vi "Max Bin transfer (single queue).vi"(11 "Enum":enum16{"1", "2", "3", "4"}(ring)) -> (1 "Next state":enum16{"1", "2", "3", "4"}(ring), 3 "END?":bool)   [LabVIEW 2014]
uses:
  <vilib>/rvi/Emulation/niFpgaEmulationIsFPGAContextNoSignature.vi
  <vilib>/rvi/DataTransferAndStorage/Container/Common/niFpgaContainerGetUniqueNameForEmu.vi
  <vilib>/rvi/Memory/Memory_Emulation/niFpgaMemoryEmulationCacheClearOnFirstRun.vi
  <vilib>/rvi/Memory/Memory_Emulation/nirvimemoryEmulationManagerCache_MakeExclusive.vi
  <vilib>/rvi/Memory/Memory_Emulation/niFpgaMemoryEmulationValidateCache.vi
  <vilib>/rvi/Memory/Memory_Emulation/nirvimemoryEmulationManagerCache_InsertValue.vi
  <vilib>/Utility/error.llb/Clear Errors.vi
  <vilib>/rvi/Memory/Memory_Emulation/nirvimemoryEmulationManagerCache_ReleaseExclusive.vi
  <vilib>/rvi/Memory/Memory_Emulation/nirvimemoryEmulationManagerCache_GetValue.vi
  <vilib>/rvi/Memory/Memory_Emulation/nirvimemoryEmulationManagerCache_SetValue.vi
  <vilib>/rvi/Emulation/niFpgaProcessEmulError.vi
  <vilib>/rvi/Emulation/niFpgaSctlEmulationGetInTimedLoop.vi
  <vilib>/rvi/interface/RandomDataEmulation/niFpgaRandomDataHandleErrors.vi
  <vilib>/rvi/DataTransferAndStorage/Container/XNode/niFpgaContainer.xnode
  <vilib>/rvi/DataTransferAndStorage/Register/Emulation/niFpgaRegisterEmulation.vi
  <vilib>/rvi/interface/RandomDataEmulation/nirviRandomDataFpgaReadWriteTemplate.vi
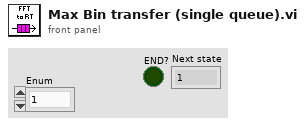
[diagram p1: front panel]
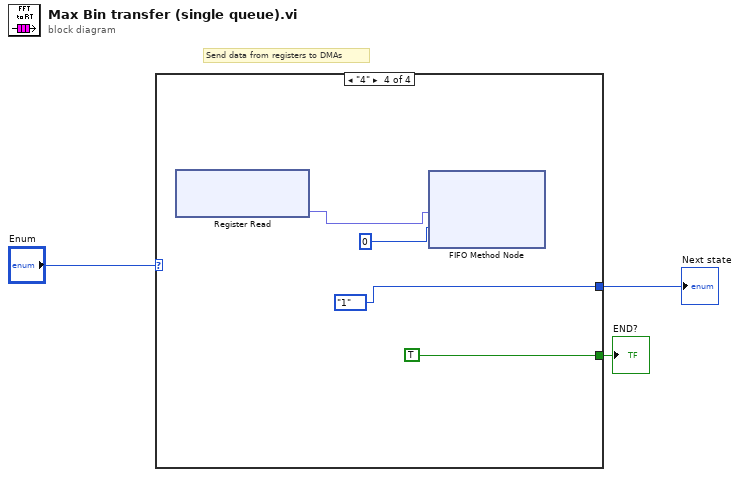
[diagram p0: block diagram]
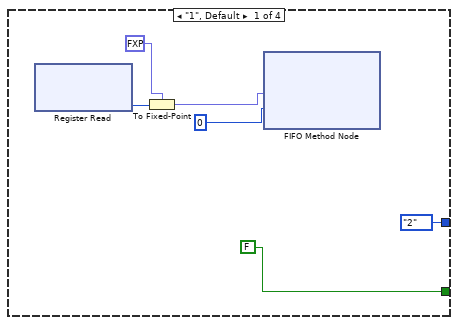
[diagram p2: hidden frame]
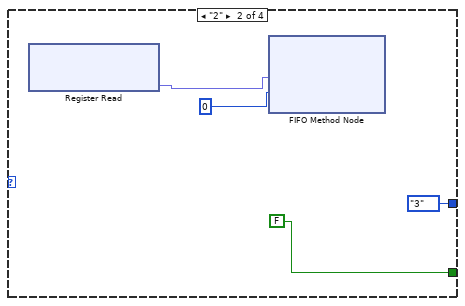
[diagram p3: hidden frame]
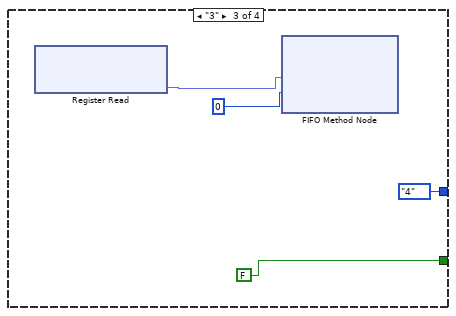
[diagram p4: hidden frame]
diagram:
  # "Send data from registers to DMAs"
  n1 = case shown="\"4\"" "Enum" {
    tunnel: [FALSE ("Timed Out?") FALSE ("Timed Out?") FALSE ("Timed Out?") TRUE ("Timed Out?")] -> w2
    tunnel: [enum16{"1", "2", "3", "4"}."2" ("Enum") enum16{"1", "2", "3", "4"}."3" ("Enum") enum16{"1", "2", "3", "4"}."4" ("Enum") enum16{"1", "2", "3", "4"}."1" ("Enum")] -> w1
    frame "1", Default {
      n2 = xnode ("Register Read")() -> ("Data"=w9:i32)  [unwired: 1 in, 1 out]
      n3 = To Fixed-Point(fixed-point type=fxp<+,44,44> 0.0 ("Data"), number=w9) -> (fixed-point=w7:fxp<+,44,44>)
      n4 = xnode ("FIFO Method Node")("Element"=w7, "Timeout"=0) -> ()  [unwired: 1 in, 2 out]
    }
    frame "2" {
      n5 = xnode ("Register Read")() -> ("Data"=w12:fxp<+,44,44>)  [unwired: 1 in, 1 out]
      n6 = xnode ("FIFO Method Node")("Element"=w12, "Timeout"=0) -> ()  [unwired: 1 in, 2 out]
    }
    frame "3" {
      n7 = xnode ("Register Read")() -> ("Data"=w16:fxp<+,44,44>)  [unwired: 1 in, 1 out]
      n8 = xnode ("FIFO Method Node")("Element"=w16, "Timeout"=0) -> ()  [unwired: 1 in, 2 out]
    }
    frame "4" {
      n9 = xnode ("Register Read")() -> ("Data"=w20:fxp<+,44,44>)  [unwired: 1 in, 1 out]
      n10 = xnode ("FIFO Method Node")("Element"=w20, "Timeout"=0) -> ()  [unwired: 1 in, 2 out]
    }
  }
  "END?" <- w2
  "Next state" <- w1
